vi "EditParam1.vi"(9 "Index":u32, 10 "type":u16(ring)=2 items=["USB-CAN"=2, "USB-CAN2.0"=3], 11 "param":T1[](array[typedef]) {"ACR0" format="%x"}) -> (1 "Channels":u32[](array[numeric]), 2 "DevIndex":u32, 3 "param out":T1[](array[typedef]) {"ACR0" format="%x"})   [LabVIEW 2011]
uses:
  Param.ctl
panel:
  in  "AllChl":bool=TRUE
  in  "DevInd":enum32{"0", "1", "2", "3", "4", "5", "6", "7"}(ring) caption="设备索引号："
  in  "Filter":u8(ring)=1 caption="滤波方式：" items=["接收所有类型"=1, "只收标准帧"=2, "只收扩展帧"=3]
  in  "Cancel":bool
  in  "OK":bool
  in  "channel":enum16{"通道1", "通道2"}(ring) caption="选择CAN通道号："
  in  "屏蔽码":u32=4294967295 caption="屏蔽码:" format="0x%08x"
  in  "验收码":u32=2147483648 caption="验收码:" format="0x%08x"
  in  "工作模式:":u16(ring) items=["正常工作", "仅监帧听模式", "自测模试（环回模式）"]
  in  "BTR1":u8=28 caption="(HEX)" format="%02x"
  in  "BTR0":u8=1 caption="BTR0/1:" format="%02x"
  in  "br":u32(ring)=8 caption="波特率:" items=["5k bps"=1, "10k bps"=2, "20k bps"=3, "40k bps"=4, "50k bps"=5, "80k bps"=6, "100k bps"=7, "125k bps"=8, "200k bps"=9, "250k bps"=10, "400k bps"=11, "500k bps"=12, "666k bps"=13, "800k bps"=14, "1000k bps"=15, "self define"=16]
  # "CAN参数"
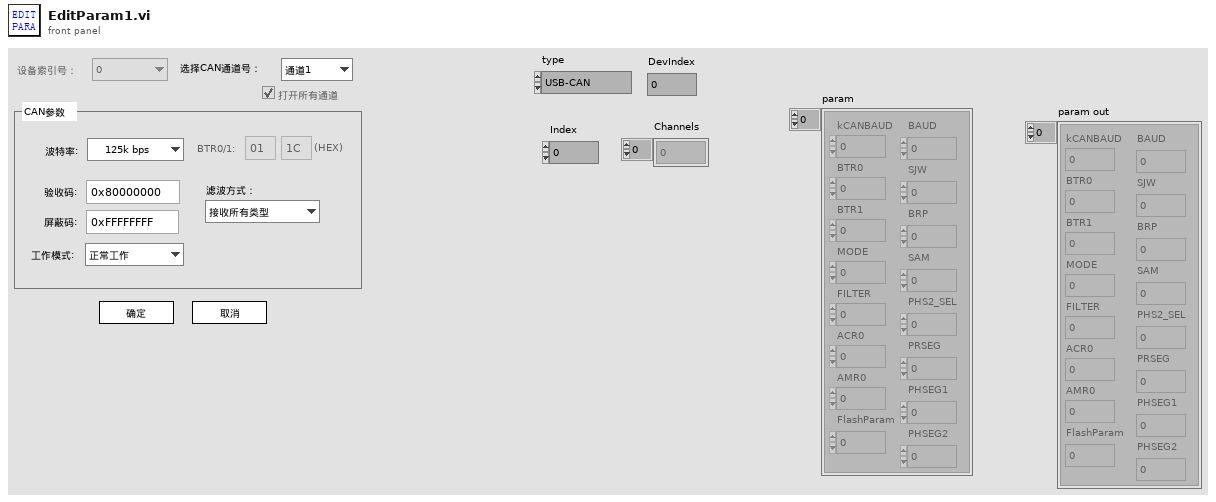
[diagram p1: front panel]
types:
  T1 = typedef "Param.ctl" = cluster{"kCANBAUD":u8, "BTR0":u8, "BTR1":u8, "MODE":u8, "FILTER":u8, "ACR0":u32, "AMR0":u32, "FlashParam":u32, "BAUD":u32, "SJW":u8, "BRP":u8, "SAM":u8, "PHS2_SEL":u8, "PRSEG":u8, "PHSEG1":u8, "PHSEG2":u8}
  T2 = enum8{"Enabled", "Disabled", "Disabled and Grayed Out"}
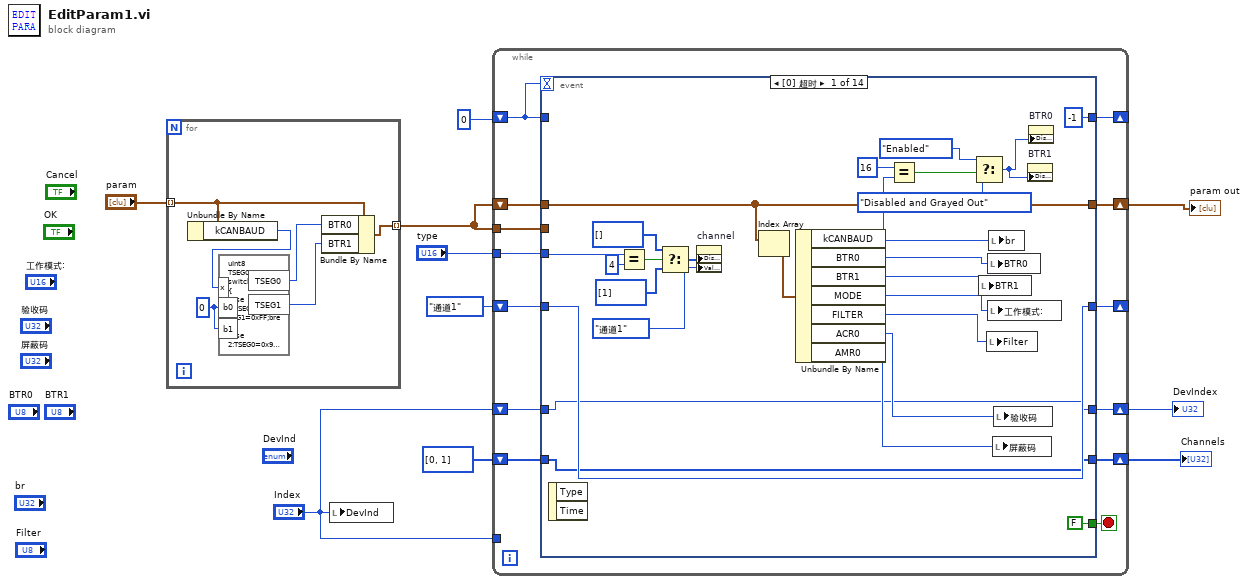
[diagram p0: block diagram]
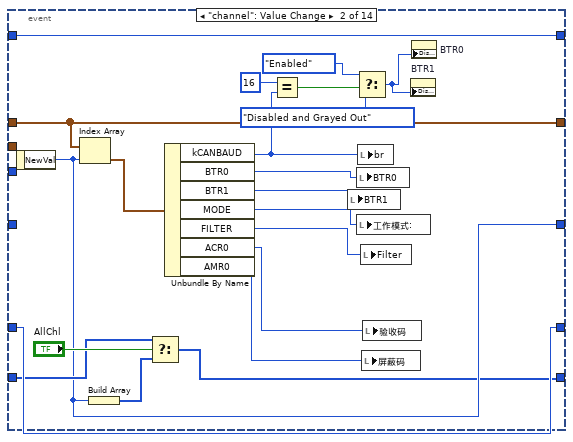
[diagram p2: hidden frame]
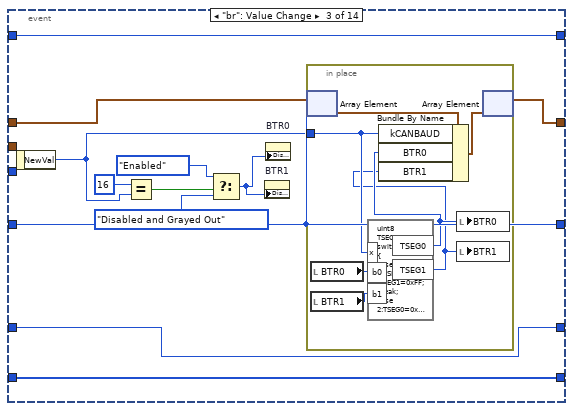
[diagram p3: hidden frame]
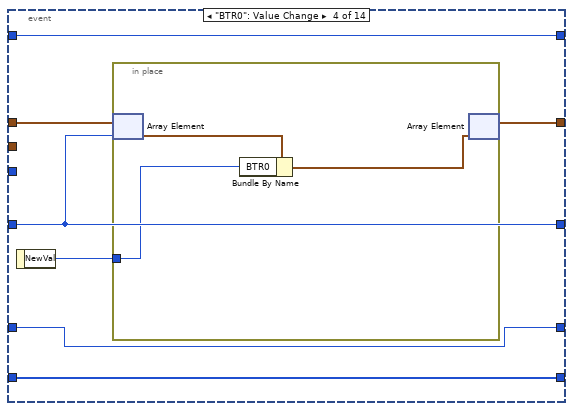
[diagram p4: hidden frame]
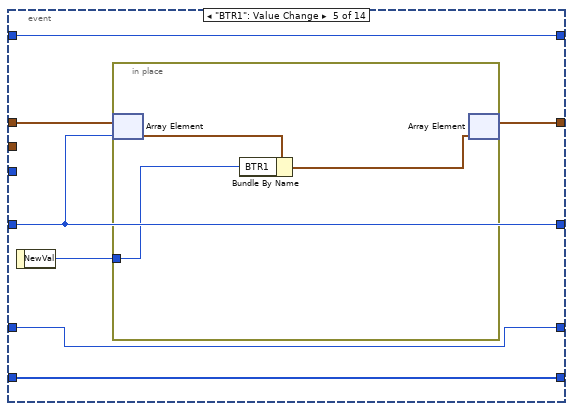
[diagram p5: hidden frame]
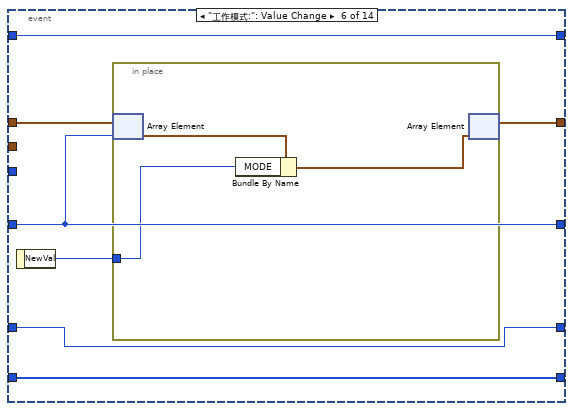
[diagram p6: hidden frame]
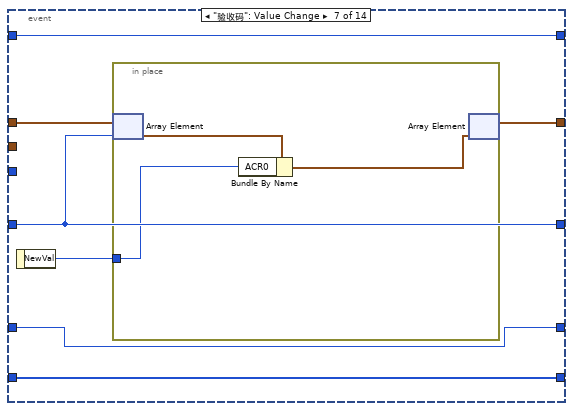
[diagram p7: hidden frame]
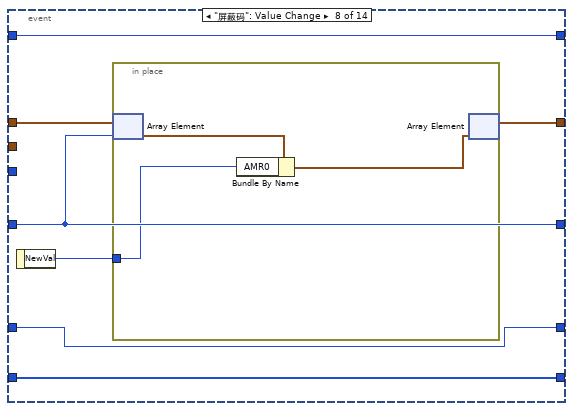
[diagram p8: hidden frame]
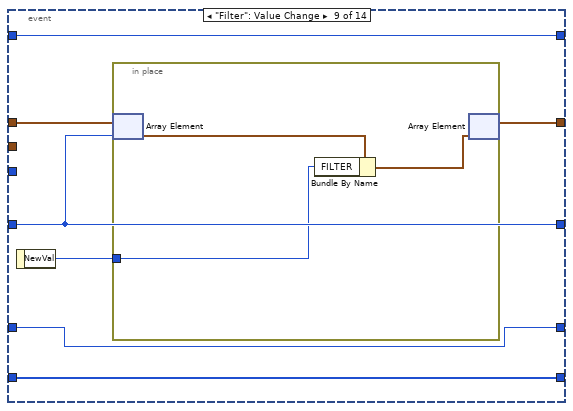
[diagram p9: hidden frame]
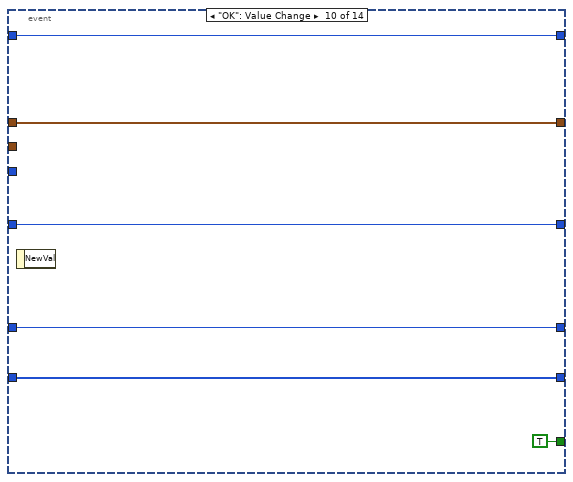
[diagram p10: hidden frame]
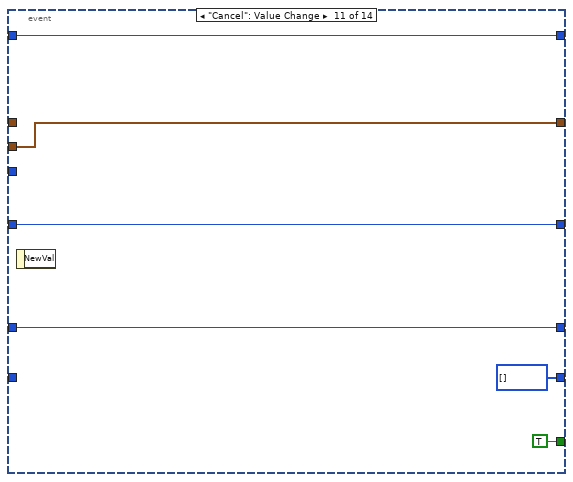
[diagram p11: hidden frame]
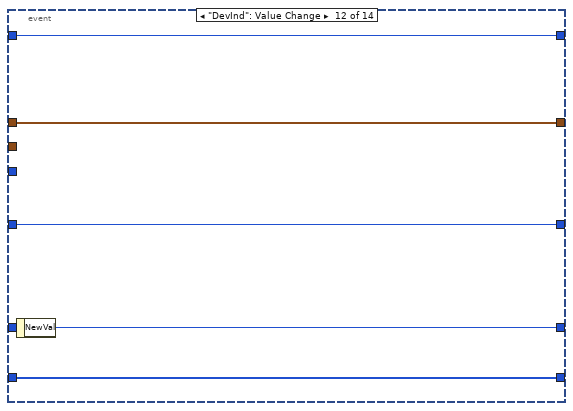
[diagram p12: hidden frame]
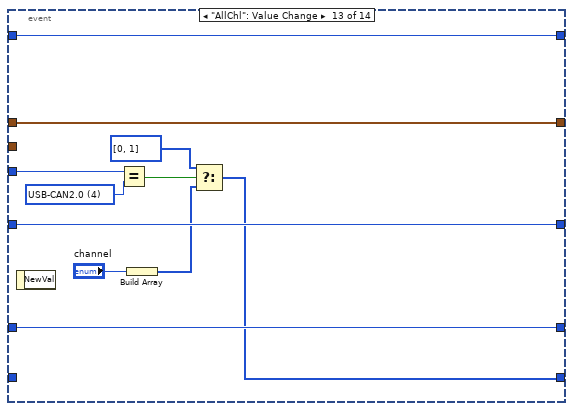
[diagram p13: hidden frame]
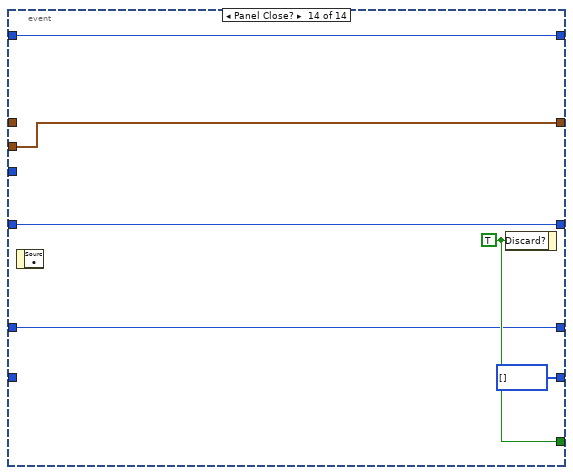
[diagram p14: hidden frame]
diagram:
  n1 = for {
    tunnel: "param" -> [w14] mode=indexing
    tunnel: [w13] -> w6 mode=indexing
    w16 = u8 0 ("输入变量")
    n2 = Unbundle By Name(w14) -> ("kCANBAUD"=w15:u8)
    n3 = formula code="uInt8 TSEG0,TSEG1;\nswitch(x)\n{ \ncase 1:TSEG0=0x9F;TSEG1=0xFF;break;\ncase 2:TSEG0=0x9F;TSEG1=0xFF;break;\ncase 3:TSEG0=0x18;TSEG1=0x1c;break;\ncase 4:TSEG0=0x87;TSEG1=0xff;break;\ncase 5:TSEG0=0x09;TSEG1=0x1c;break;\ncase 6:TSEG0=0x83;TSEG1=0xff;break;\ncase 7:TSEG0=0x04;TSEG1=0x1c;break;\ncase 8:TSEG0=0x03;TSEG1=0x1c;break;\ncase 9:TSEG0=0x81;TSEG1=0xfa;break;\ncase 10:TSEG0=0x01;TSEG1=0x1c;break;\ncase 11:TSEG0=0x80;TSEG1=0xfa;break;\ncase 12:TSEG0=0x00;TSEG1=0x1c;break;\ncase 13:TSEG0=0x80;TSEG1=0xb6;break;\ncase 14:TSEG0=0x00;TSEG1=0x16;break;\ncase 15:TSEG0=0x00;TSEG1=0x14;break;\ndefault:TSEG0=b0;TSEG1=b1;\n}"("x"=w15, "b0"=w16, "b1"=w16) -> ("TSEG0"=w12:u8, "TSEG1"=w11:u8)
    n4 = Bundle By Name(cluster=w14, "BTR0"=w12, "BTR1"=w11) -> (w13:T1)
  }
  n5 = local write "DevInd"("Index") -> ()
  n6 = while {
    shift-right: [w27] -> w8
    shift-left: w6 -> [w28]
    shift-right: [w26] -> _
    shift-left: 0 -> [w25]
    tunnel: "type" -> [w24]
    shift-right: [w23] -> _
    shift-left: enum16{"通道1", "通道2"}."通道1" ("NewVal") -> [w22]
    tunnel: w6 -> [w21]
    shift-right: [w19] -> w5
    shift-left: "Index" -> [w20]
    shift-right: [w17] -> w3
    shift-left: u32[] [0, 1] ("Channels") -> [w18]
    tunnel: "Index" -> [_]
    stop <- w29 stop-if-true
    n7 = event shown="[0] 超时" {
      selector: _ -> [_ _ _ _ _ _ _ _ _ _ _ _ _ _]
      dyn-events: _ -> [_ _ _ _ _ _ _ _ _ _ _ _ _ _]
      timeout: w25 -> [_ _ _ _ _ _ _ _ _ _ _ _ _ _]
      tunnel: [FALSE _ _ _ _ _ _ _ _ TRUE TRUE _ _ w187] -> w29
      tunnel: w28 -> [w46 w75 w82 w101 w111 w121 w131 w141 w151 w161 _ w172 w183 _]
      tunnel: [w46 w75 w80 w99 w109 w119 w129 w139 w150 w161 w164 w172 w183 w186] -> w27
      tunnel: [-1 w76 w88 w102 w112 w122 w132 w142 w152 w160 w167 w171 w182 w189] -> w26
      tunnel: w25 -> [_ w76 w88 w102 w112 w122 w132 w142 w152 w160 w167 w171 w182 w189]
      tunnel: w24 -> [w53 _ _ _ _ _ _ _ _ _ _ _ w179 _]
      tunnel: [w33 w58 w81 w98 w108 w118 w128 w138 w149 w159 w166 w170 w181 w188] -> w23
      tunnel: w22 -> [w33 _ w81 w98 w108 w118 w128 w138 w149 w159 w166 w170 w181 w188]
      tunnel: w21 -> [_ _ _ _ _ _ _ _ _ _ w164 _ _ w186]
      tunnel: w20 -> [w31 w61 w78 w97 w107 w117 w127 w137 w147 w157 w163 _ w180 w185]
      tunnel: [w31 w61 w78 w97 w107 w117 w127 w137 w147 w157 w163 w169 w180 w185] -> w19
      tunnel: w18 -> [w30 w59 w77 w96 w106 w116 w126 w136 w146 w156 _ w168 _ _]
      tunnel: [w30 w56 w77 w96 w106 w116 w126 w136 w146 w156 u32[] [] ("Channels") w168 w173 u32[] [] ("Channels")] -> w17
      event Timeout {
        n8 = event-data() -> ()  [unwired: 1 in, 2 out]
        n9 = Equal?(x=w53, y=u16 4) -> (x = y?=w51:bool)
        n10 = Select(t=i32[] [] ("禁用项[]"), s=w51, f=i32[] [1] ("禁用项[]")) -> (s? t:f=w48:i32[])
        n11 = property on="channel" class="Enum (严格)"("Disabled Items []"=w48, "Value"=enum16{"通道1", "通道2"}."通道1" ("channel")) -> ()  [unwired: 2 in, 2 out]
        n12 = Index Array(array=w46) -> (element=w45:T1)  [unwired: 1 in]
        n13 = Unbundle By Name(w45) -> ("kCANBAUD"=w39:u8, "BTR0"=w44:u8, "BTR1"=w43:u8, "MODE"=w42:u8, "FILTER"=w32:u8, "ACR0"=w41:u32, "AMR0"=w40:u32)
        n14 = Equal?(x=u8 16, y=w39) -> (x = y?=w35:bool)
        n15 = Select(t=T2."Enabled" ("禁用"), s=w35, f=T2."Disabled and Grayed Out") -> (s? t:f=w34:T2)
        n16 = local write "BTR1"(w43) -> ()
        n17 = local write "Filter"(w32) -> ()
        n18 = local write "BTR0"(w44) -> ()
        n19 = local write "工作模式:"(w42) -> ()
        n20 = local write "br"(w39) -> ()
        n21 = local write "屏蔽码"(w40) -> ()
        n22 = local write "验收码"(w41) -> ()
        n23 = property on="BTR1" class="DigNum (严格)"("DisabledEnum"=w34) -> ()  [unwired: 2 in, 2 out]
        n24 = property on="BTR0" class="DigNum (严格)"("DisabledEnum"=w34) -> ()  [unwired: 2 in, 2 out]
      }
      event "channel": Value Change {
        n25 = event-data() -> ("NewVal"=w58:enum16{"通道1", "通道2"})  [unwired: 1 in]
        n26 = Index Array(array=w75, index=w58) -> (element=w69:T1)
        n27 = Build Array(w58) -> (w57:enum16{"通道1", "通道2"}[])
        n28 = Select(t=w59, s="AllChl", f=w57) -> (s? t:f=w56:u32[])
        n29 = Unbundle By Name(w69) -> ("kCANBAUD"=w63:u8, "BTR0"=w74:u8, "BTR1"=w73:u8, "MODE"=w72:u8, "FILTER"=w62:u8, "ACR0"=w71:u32, "AMR0"=w70:u32)
        n30 = Equal?(x=u8 16, y=w63) -> (x = y?=w65:bool)
        n31 = local write "BTR1"(w73) -> ()
        n32 = Select(t=T2."Enabled" ("禁用"), s=w65, f=T2."Disabled and Grayed Out") -> (s? t:f=w64:T2)
        n33 = local write "BTR0"(w74) -> ()
        n34 = local write "工作模式:"(w72) -> ()
        n35 = local write "br"(w63) -> ()
        n36 = local write "Filter"(w62) -> ()
        n37 = local write "屏蔽码"(w70) -> ()
        n38 = local write "验收码"(w71) -> ()
        n39 = property on="BTR1" class="DigNum (严格)"("DisabledEnum"=w64) -> ()  [unwired: 2 in, 2 out]
        n40 = property on="BTR0" class="DigNum (严格)"("DisabledEnum"=w64) -> ()  [unwired: 2 in, 2 out]
      }
      event "br": Value Change {
        n41 = event-data() -> ("NewVal"=w79:u32)  [unwired: 1 in]
        n42 = Equal?(x=u8 16, y=w79) -> (x = y?=w86:bool)
        n43 = Select(t=T2."Enabled" ("禁用"), s=w86, f=T2."Disabled and Grayed Out") -> (s? t:f=w85:T2)
        n44 = property on="BTR1" class="DigNum (严格)"("DisabledEnum"=w85) -> ()  [unwired: 2 in, 2 out]
        n45 = property on="BTR0" class="DigNum (严格)"("DisabledEnum"=w85) -> ()  [unwired: 2 in, 2 out]
        n46 = in-place {
          in-place-border: w79 -> [w93]
          n47 = in-place-array #1(w82, w81) -> (w95:T1)
          n48 = local read "BTR0"() -> (w90:u8)
          n49 = local read "BTR1"() -> (w89:u8)
          n50 = formula code="uInt8 TSEG0,TSEG1;\nswitch(x)\n{ \ncase 1:TSEG0=0x9F;TSEG1=0xFF;break;\ncase 2:TSEG0=0x9F;TSEG1=0xFF;break;\ncase 3:TSEG0=0x18;TSEG1=0x1c;break;\ncase 4:TSEG0=0x87;TSEG1=0xff;break;\ncase 5:TSEG0=0x09;TSEG1=0x1c;break;\ncase 6:TSEG0=0x83;TSEG1=0xff;break;\ncase 7:TSEG0=0x04;TSEG1=0x1c;break;\ncase 8:TSEG0=0x03;TSEG1=0x1c;break;\ncase 9:TSEG0=0x81;TSEG1=0xfa;break;\ncase 10:TSEG0=0x01;TSEG1=0x1c;break;\ncase 11:TSEG0=0x80;TSEG1=0xfa;break;\ncase 12:TSEG0=0x00;TSEG1=0x1c;break;\ncase 13:TSEG0=0x80;TSEG1=0xb6;break;\ncase 14:TSEG0=0x00;TSEG1=0x16;break;\ncase 15:TSEG0=0x00;TSEG1=0x14;break;\ndefault:TSEG0=b0;TSEG1=b1;\n}"("x"=w93, "b0"=w90, "b1"=w89) -> ("TSEG0"=w92:u8, "TSEG1"=w91:u8)
          n51 = Bundle By Name(cluster=w95, "kCANBAUD"=w93, "BTR0"=w92, "BTR1"=w91) -> (w94:T1)
          n52 = local write "BTR0"(w92) -> ()
          n53 = local write "BTR1"(w91) -> ()
          n54 = in-place-array #1(w94) -> (w80:T1[])  [unwired: 1 out]
        }
      }
      event "BTR0": Value Change {
        n55 = event-data() -> ("NewVal"=w100:u8)  [unwired: 1 in]
        n56 = in-place {
          in-place-border: w100 -> [w104]
          n57 = in-place-array #2(w101, w98) -> (w105:T1)
          n58 = Bundle By Name(cluster=w105, "BTR0"=w104) -> (w103:T1)
          n59 = in-place-array #2(w103) -> (w99:T1[])  [unwired: 1 out]
        }
      }
      event "BTR1": Value Change {
        n60 = event-data() -> ("NewVal"=w110:u8)  [unwired: 1 in]
        n61 = in-place {
          in-place-border: w110 -> [w114]
          n62 = in-place-array #3(w111, w108) -> (w115:T1)
          n63 = Bundle By Name(cluster=w115, "BTR1"=w114) -> (w113:T1)
          n64 = in-place-array #3(w113) -> (w109:T1[])  [unwired: 1 out]
        }
      }
      event "工作模式:": Value Change {
        n65 = event-data() -> ("NewVal"=w120:u16)  [unwired: 1 in]
        n66 = in-place {
          in-place-border: w120 -> [w124]
          n67 = in-place-array #4(w121, w118) -> (w125:T1)
          n68 = Bundle By Name(cluster=w125, "MODE"=w124) -> (w123:T1)
          n69 = in-place-array #4(w123) -> (w119:T1[])  [unwired: 1 out]
        }
      }
      event "验收码": Value Change {
        n70 = event-data() -> ("NewVal"=w130:u32)  [unwired: 1 in]
        n71 = in-place {
          in-place-border: w130 -> [w134]
          n72 = in-place-array #5(w131, w128) -> (w135:T1)
          n73 = Bundle By Name(cluster=w135, "ACR0"=w134) -> (w133:T1)
          n74 = in-place-array #5(w133) -> (w129:T1[])  [unwired: 1 out]
        }
      }
      event "屏蔽码": Value Change {
        n75 = event-data() -> ("NewVal"=w140:u32)  [unwired: 1 in]
        n76 = in-place {
          in-place-border: w140 -> [w144]
          n77 = in-place-array #6(w141, w138) -> (w145:T1)
          n78 = Bundle By Name(cluster=w145, "AMR0"=w144) -> (w143:T1)
          n79 = in-place-array #6(w143) -> (w139:T1[])  [unwired: 1 out]
        }
      }
      event "Filter": Value Change {
        n80 = event-data() -> ("NewVal"=w148:u8)  [unwired: 1 in]
        n81 = in-place {
          in-place-border: w148 -> [w153]
          n82 = in-place-array #7(w151, w149) -> (w155:T1)
          n83 = Bundle By Name(cluster=w155, "FILTER"=w153) -> (w154:T1)
          n84 = in-place-array #7(w154) -> (w150:T1[])  [unwired: 1 out]
        }
      }
      event "OK": Value Change {
        n85 = event-data() -> ()  [unwired: 1 in, 1 out]
      }
      event "Cancel": Value Change {
        n86 = event-data() -> ()  [unwired: 1 in, 1 out]
      }
      event "DevInd": Value Change {
        n87 = event-data() -> ("NewVal"=w169:enum32{"0", "1", "2", "3", "4", "5", "6", "7"})  [unwired: 1 in]
      }
      event "AllChl": Value Change {
        w178 = u16 4 items=["USB-CAN"=3, "USB-CAN2.0"=4] ("type")
        n88 = event-data() -> ()  [unwired: 1 in, 1 out]
        n89 = Equal?(x=w179, y=w178) -> (x = y?=w177:bool)
        n90 = Build Array("channel") -> (w174:enum16{"通道1", "通道2"}[])
        n91 = Select(t=u32[] [0, 1] ("Channels"), s=w177, f=w174) -> (s? t:f=w173:u32[])
      }
      event Panel Close? {
        w187 = TRUE ("放弃？")
        n92 = event-data() -> ()  [unwired: 1 in, 1 out]
        n93 = event-data("Discard?"=w187) -> ()  [unwired: 1 in, 1 out]
      }
    }
  }
  "param out" <- w8
  "DevIndex" <- w5
  "Channels" <- w3
